vi "data_log_right.vi"(9 "Path Selected":string, 10 "Data to Log":i32[](array[numeric]), 11 "NXT/EV3 In":T1) -> (3 "NXT/EV3 Out":T1)   [LabVIEW 2012, in "Serenity_mk2.lvrbt"]
uses:
  Serenity_mk2.lvrbt
  <vilib>/NXT/Subs/LVHSConnector.ctl
  <vilib>/NXT/LegoClasses/BrickReference/BrickReference.lvclass
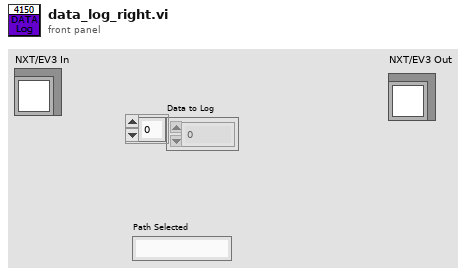
[diagram p1: front panel]
types:
  T1 = typedef "LVHSConnector.ctl" = refnum<class "BrickReference.lvclass">
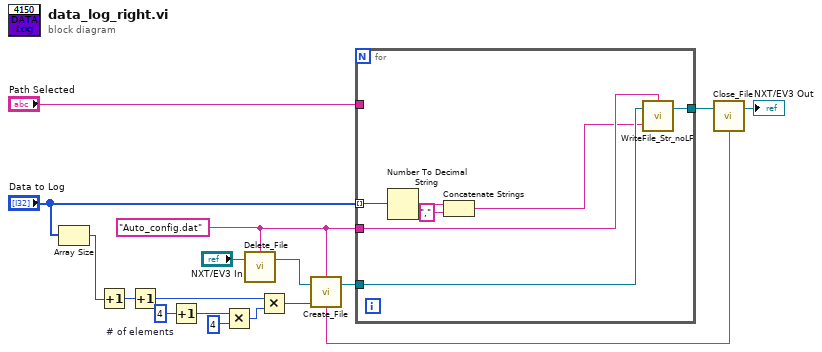
[diagram p0: block diagram]
diagram:
  w13 = 4  # # of elements
  w3 = "Auto_config.dat" ("Filename")
  n1 = Array Size(array="Data to Log") -> (size(s)=w6:i32)
  n2 = Increment(x=w6) -> (x+1=w14:i32)
  n3 = Increment(x=w14) -> (x+1=w9:i32)
  n4 = Increment(x=w13) -> (x+1=w12:i32)
  n5 = Multiply(x=w12, y=u32 4) -> (x*y=w11:u32)
  n6 = call <vilib>:"Delete_File.vi"("NXT/EV3"="NXT/EV3 In", "Filename"=w3) -> ("NXT/EV3"=w8:T1)  [unwired: 2 in]
  n7 = Multiply(x=w9, y=w11) -> (x*y=w15:u32)
  n8 = call <vilib>:"Create_File.vi"("File Size (256)"=w15, "NXT/EV3"=w8, "Filename"=w3) -> ("NXT/EV3"=w5:T1)  [unwired: 1 out]
  n9 = for {
    tunnel: "Path Selected" -> [_]
    tunnel: "Data to Log" -> [w21] mode=indexing
    tunnel: w5 -> [w23]
    tunnel: w3 -> [w20]
    tunnel: [w22] -> w4
    n10 = Number To Decimal String(number=w21) -> (decimal integer string=w19:string)  [unwired: 1 in]
    n11 = Concatenate Strings(w19, "," ("string")) -> (w18:string)
    n12 = call <vilib>:"WriteFile_Str_noLF.vi"("String"=w18, "NXT/EV3"=w23, "Filename"=w20) -> ("NXT/EV3"=w22:T1)  [unwired: 1 in]
  }
  n13 = call <vilib>:"Close_File.vi"("NXT/EV3"=w4, "Filename"=w3) -> ("NXT/EV3"=→"NXT/EV3 Out":T1)  [unwired: 2 in]
